vi "北斗参数配置.vi"() -> ()   [LabVIEW 2016, in "环境动力监测库.lvlib" / "NMEA.lvlib"]
uses:
  NMEA.lvlib
panel:
  in  "收方地址设定值":string
  in  "移位报警设定值":dbl=1000.0
  # "北斗参数配置"
  # "米"
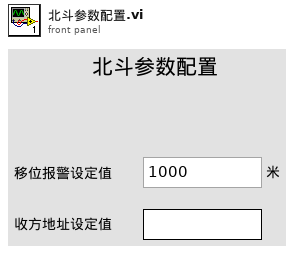
[diagram p1: front panel]
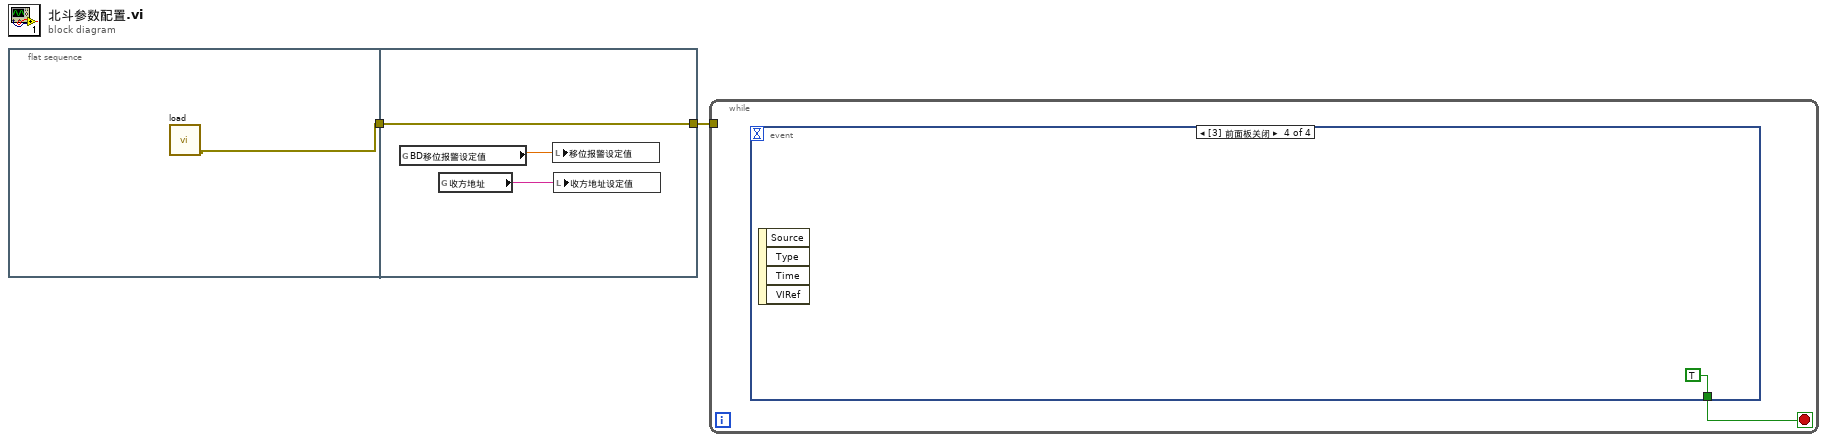
[diagram p0: block diagram]
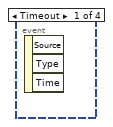
[diagram p2: hidden frame]
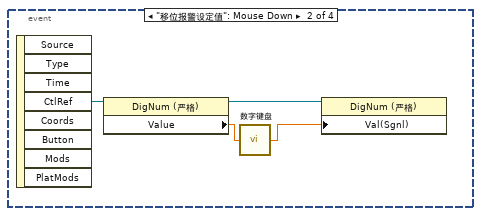
[diagram p3: hidden frame]
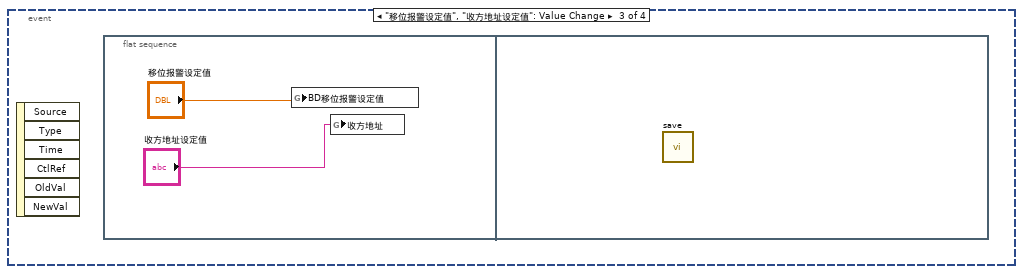
[diagram p4: hidden frame]
diagram:
  n1 = flat-sequence {
    tunnel: [w3] -> w2
    tunnel: [w6] -> w1
    tunnel: w2 -> [w6]
    frame #0 {
      n2 = call "load.vi"() -> ("error out"=w3:errorcluster)  [unwired: 11 in]
    }
    frame #1 {
      n3 = global read "断电保存全局变量.vi" "BD移位报警设定值"() -> (w4:dbl)
      n4 = global read "断电保存全局变量.vi" "收方地址"() -> (w5:string)
      n5 = local write "移位报警设定值"(w4) -> ()
      n6 = local write "收方地址设定值"(w5) -> ()
    }
  }
  n7 = while {
    tunnel: w1 -> [_]
    stop <- w7 stop-if-true
    n8 = event shown="[3] 前面板关闭" {
      selector: _ -> [_ _ _ _]
      dyn-events: _ -> [_ _ _ _]
      timeout: _ -> [_ _ _ _]
      tunnel: [_ _ _ TRUE] -> w7
      event Timeout {
        n9 = event-data() -> ()  [unwired: 1 in, 3 out]
      }
      event "移位报警设定值": Mouse Down {
        n10 = event-data() -> ("CtlRef"=w8:refnum<vi>)  [unwired: 1 in, 7 out]
        n11 = property class="DigNum (严格)"(reference=w8) -> (reference out=w10:refnum<vi>, "Value"=w11:dbl)  [unwired: 1 in, 1 out]
        n12 = call "数字键盘.vi"("OldNumber"=w11) -> ("NewNumber"=w9:sgl)
        n13 = property class="DigNum (严格)"(reference=w10, "Val(Sgnl)"=w9) -> ()  [unwired: 1 in, 2 out]
      }
      event "移位报警设定值", "收方地址设定值": Value Change {
        n14 = event-data() -> ()  [unwired: 1 in, 6 out]
        n15 = flat-sequence {
          frame #0 {
            n16 = global write "断电保存全局变量.vi" "BD移位报警设定值"("移位报警设定值") -> ()
            n17 = global write "断电保存全局变量.vi" "收方地址"("收方地址设定值") -> ()
          }
          frame #1 {
            n18 = call "save.vi"() -> ()  [unwired: 11 in, 1 out]
          }
        }
      }
      event Panel Close {
        n19 = event-data() -> ()  [unwired: 1 in, 4 out]
      }
    }
  }
